vi "visa1.vi"() -> ()   [LabVIEW 2015]
uses:
  <vilib>/Instr/_visa.llb/VISA Configure Serial Port (Instr).vi
panel:
  out "output array":string[](array[string])
  out "LDR  2":string
  in  "stop":bool
  out "LDR 1":string
  out "read buffer":string
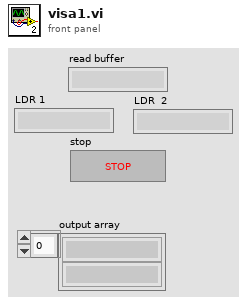
[diagram p1: front panel]
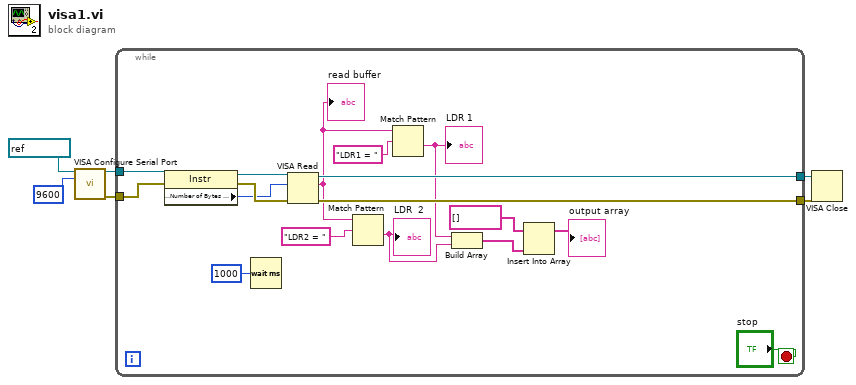
[diagram p0: block diagram]
diagram:
  n1 = call-poly "VISA Configure Serial Port"("VISA resource name"=refnum<visa-resource-name> "COM4", "baud rate (9600)"=u32 9600) -> ("VISA resource name out"=w6:refnum<visa-resource-name>, "error out"=w5:errorcluster)  [unwired: 12 in]
  n2 = while {
    tunnel: w6 -> [w23]
    tunnel: w5 -> [w22]
    tunnel: [w18] -> w4
    tunnel: [w17] -> w3
    stop <- "stop" stop-if-true
    n3 = property class="Instr"(reference=w23, error in=w22) -> (reference out=w19:refnum<visa-resource-name>, error out=w21:errorcluster, "Serial Settings:Number of Bytes at Serial Port"=w20:u32)
    n4 = Wait (ms)(milliseconds to wait=u32 1000) -> ()  [unwired: 1 out]
    n5 = VISA Read(VISA resource name=w19, byte count=w20, error in (no error)=w21) -> (VISA resource name out=w18:refnum<visa-resource-name>, read buffer=w7:string, error out=w17:errorcluster)  [unwired: 1 out]
    "read buffer" <- w7
    n6 = Match Pattern(string=w7, regular expression="LDR2 = ") -> (after substring=w11:string)  [unwired: 1 in, 3 out]
    "LDR  2" <- w11
    n7 = Match Pattern(string=w7, regular expression="LDR1 = ") -> (after substring=w12:string)  [unwired: 1 in, 3 out]
    "LDR 1" <- w12
    n8 = Build Array(w12, w11) -> (w10:string[])
    n9 = Insert Into Array(array=string[] [], new element=w10) -> (→"output array":string[])  [unwired: 1 in]
  }
  n10 = VISA Close(VISA resource name=w4, error in (no error)=w3) -> ()  [unwired: 1 out]
